vi "Close.vi"(8 "error in":errorcluster, 11 "Parallel Mode Channels in":refnum<class "Parallel Mode Channels.lvclass">) -> (0 "error out":errorcluster, 3 "Parallel Mode Channels out":refnum<class "Parallel Mode Channels.lvclass">)   [LabVIEW 2023, in "Parallel Mode Channels.lvclass"]
uses:
  Parallel Mode Channels.lvclass
  <vilib>/ADAS Replay HIL/AdasHilServices/AdasHilChannelServices.lvlib
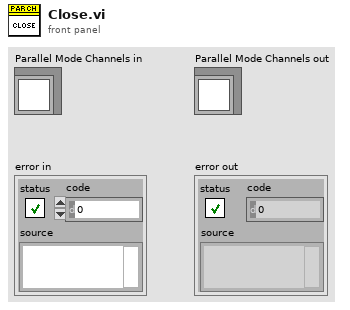
[diagram p1: front panel]
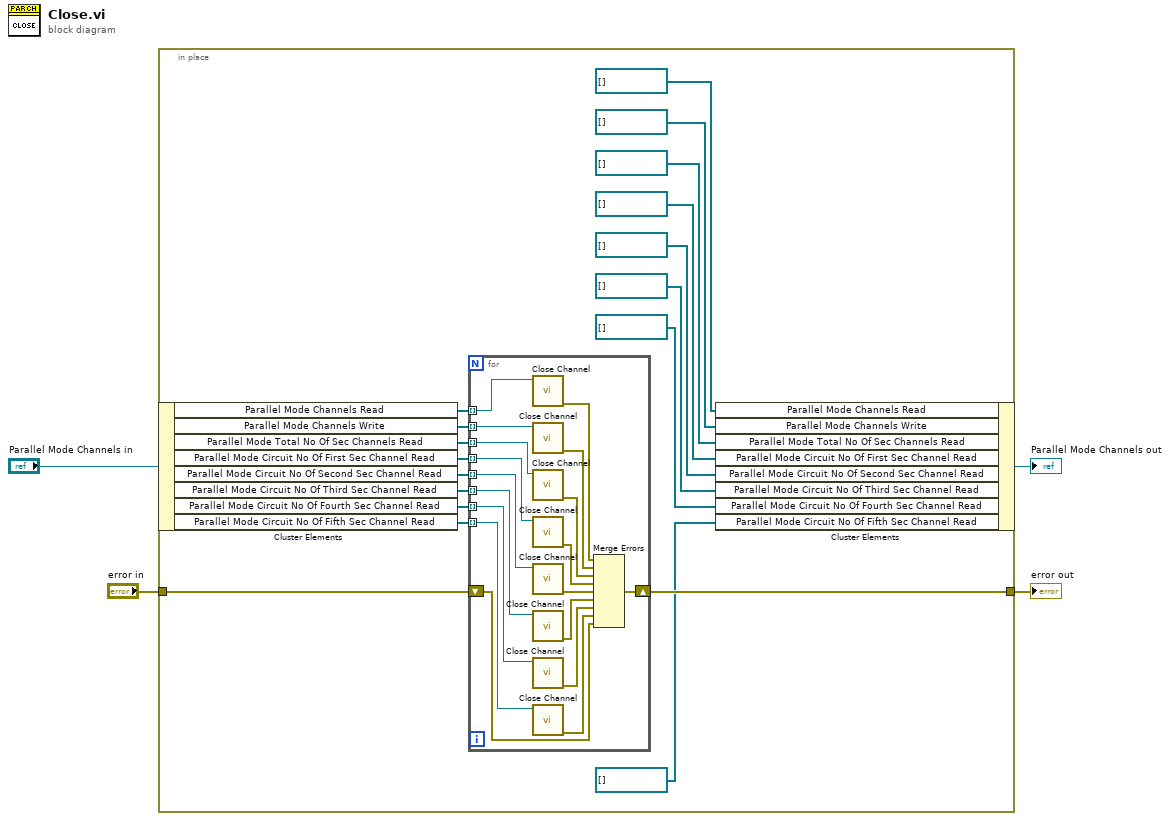
[diagram p0: block diagram]
diagram:
  n1 = in-place {
    in-place-border: "error in" -> [w22]
    in-place-border: [w21] -> w1
    n2 = in-place-cluster #1("Parallel Mode Channels in") -> ("Parallel Mode Channels Read"=w20:refnum<k21>[], "Parallel Mode Channels Write"=w19:refnum<k21>[], "Parallel Mode Total No Of Sec Channels Read"=w16:refnum<k21>[], "Parallel Mode Circuit No Of First Sec Channel Read"=w15:refnum<k21>[], "Parallel Mode Circuit No Of Second Sec Channel Read"=w14:refnum<k21>[], "Parallel Mode Circuit No Of Third Sec Channel Read"=w13:refnum<k21>[], "Parallel Mode Circuit No Of Fourth Sec Channel Read"=w12:refnum<k21>[], "Parallel Mode Circuit No Of Fifth Sec Channel Read"=w11:refnum<k21>[])
    n3 = for {
      tunnel: w20 -> [w40] mode=indexing
      tunnel: w19 -> [w39] mode=indexing
      shift-right: [w38] -> w21
      shift-left: w22 -> [w23]
      tunnel: w16 -> [w34] mode=indexing
      tunnel: w15 -> [w32] mode=indexing
      tunnel: w14 -> [w30] mode=indexing
      tunnel: w13 -> [w28] mode=indexing
      tunnel: w12 -> [w27] mode=indexing
      tunnel: w11 -> [w25] mode=indexing
      n4 = call <vilib>:"Close Channel.vi"("ADAS HIL Channel"=w40) -> ("error out"=w37:errorcluster)  [unwired: 10 in]
      n5 = call <vilib>:"Close Channel.vi"("ADAS HIL Channel"=w39) -> ("error out"=w36:errorcluster)  [unwired: 10 in]
      n6 = call <vilib>:"Close Channel.vi"("ADAS HIL Channel"=w34) -> ("error out"=w35:errorcluster)  [unwired: 10 in]
      n7 = call <vilib>:"Close Channel.vi"("ADAS HIL Channel"=w32) -> ("error out"=w33:errorcluster)  [unwired: 10 in]
      n8 = call <vilib>:"Close Channel.vi"("ADAS HIL Channel"=w30) -> ("error out"=w31:errorcluster)  [unwired: 10 in]
      n9 = call <vilib>:"Close Channel.vi"("ADAS HIL Channel"=w28) -> ("error out"=w29:errorcluster)  [unwired: 10 in]
      n10 = call <vilib>:"Close Channel.vi"("ADAS HIL Channel"=w27) -> ("error out"=w26:errorcluster)  [unwired: 10 in]
      n11 = call <vilib>:"Close Channel.vi"("ADAS HIL Channel"=w25) -> ("error out"=w24:errorcluster)  [unwired: 10 in]
      n12 = Merge Errors(w37, w36, w35, w33, w31, w29, w26, w24, w23) -> (w38:errorcluster)
    }
    n13 = in-place-cluster #1("Parallel Mode Channels Read"=refnum<k21>[] [] ("Control Mode Read"), "Parallel Mode Channels Write"=refnum<k21>[] [] ("Control Mode Read"), "Parallel Mode Total No Of Sec Channels Read"=refnum<k21>[] [], "Parallel Mode Circuit No Of First Sec Channel Read"=refnum<k21>[] [], "Parallel Mode Circuit No Of Second Sec Channel Read"=refnum<k21>[] [], "Parallel Mode Circuit No Of Third Sec Channel Read"=refnum<k21>[] [], "Parallel Mode Circuit No Of Fourth Sec Channel Read"=refnum<k21>[] [], "Parallel Mode Circuit No Of Fifth Sec Channel Read"=refnum<k21>[] []) -> (→"Parallel Mode Channels out":refnum<class "Parallel Mode Channels.lvclass">)
  }
  "error out" <- w1
